vi "Close RT FIFOs (STM Multi-Client).vi"(8 "error in (no error)":errorcluster, 11 "FIFOs In":T1 {"Data FIFO"."type" format="%0.2f"}) -> (0 "error out":errorcluster)   [LabVIEW 2016]
uses:
  <vilib>/real-time/rtfifo.llb/RTFIFORefnum DBLA.ctl
  <vilib>/real-time/rtfifo.llb/RTFIFORefnum BOOL.ctl
  RT FIFOs (STM Multi-Client).ctl
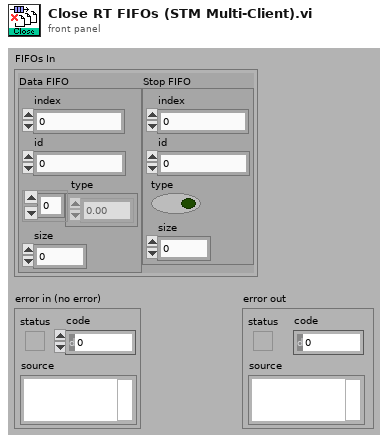
[diagram p1: front panel]
types:
  T1 = typedef "RT FIFOs (STM Multi-Client).ctl" = cluster{"Data FIFO":T2, "Stop FIFO":T3}
  T2 = typedef "NI_Real-Time Libraries.lvlib/RTFIFORefnum DBLA.ctl" = cluster{"index":u32, "id":u32, "type":dbl[], "size":u32}
  T3 = typedef "NI_Real-Time Libraries.lvlib/RTFIFORefnum BOOL.ctl" = cluster{"index":u32, "id":u32, "type":bool, "size":u32}
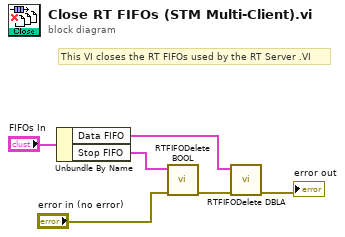
[diagram p0: block diagram]
diagram:
  # "This VI closes the RT FIFOs used by the RT Server .VI"
  n1 = Unbundle By Name("FIFOs In") -> ("Data FIFO"=w1:T2, "Stop FIFO"=w5:T3)
  n2 = call <vilib>:"RTFIFODelete BOOL.vi"("error in (no error)"="error in (no error)", "rt fifo"=w5) -> ("error out"=w3:errorcluster)  [unwired: 9 in]
  n3 = call <vilib>:"RTFIFODelete DBLA.vi"("error in (no error)"=w3, "rt fifo"=w1) -> ("error out"=→"error out":errorcluster)  [unwired: 9 in]
